vi "Data_raw-save.vi"(5 "timedelay":dbl[](array[numeric])=[0.0, 1.0, 2.0, 3.0, 4.0, 5.0, 6.0, 7.0, 8.0, 9.0], 6 "data value reference":refnum<data-value>, 7 "wavelength":dbl[](array[numeric])=[10.0, 20.0, 0.0, 0.0, 0.0, 0.0, 0.0, 0.0, 0.0, 0.0, 0.0, 0.0, 0.0, 0.0, 0.0, 0.0, 0.0, 0.0, 0.0, 0.0, 0.0, 0.0, 0.0, 0.0, 0.0, 0.0, 0.0, 0.0, 0.0, 0.0, 0.0, 0.0, 0.0, 0.0, 0.0, 0.0, 0.0, 0.0, 0.0, 0.0, 0.0, 0.0, 0.0, 0.0, 0.0, 0.0, 0.0, 0.0, 0.0, 0.0, 0.0, 0.0, 0.0, 0.0, 0.0, 0.0, 0.0, 0.0, 0.0, 0.0, 0.0, 0.0, 0.0, 0.0, 0.0, 0.0, 0.0, 0.0, 0.0, 0.0, 0.0, 0.0, 0.0, 0.0, 0.0, 0.0, 0.0, 0.0, 0.0, 0.0, 0.0, 0.0, 0.0, 0.0, 0.0, 0.0, 0.0, 0.0, 0.0, 0.0, 0.0, 0.0, 0.0, 0.0, 0.0, 0.0, 0.0, 0.0, 0.0, 100.0], 8 "error in":errorcluster, 9 "file (use dialog)":path=path "C:/Users/Sergey Denisov/Documents/REPS/TRANCON/test2.txt.txt", 10 "accuracy":string="%#g", 11 "Data raw":i32[][][][](array[numeric])) -> (0 "error out":errorcluster)   [LabVIEW 2015]
panel:
  out "Done":bool
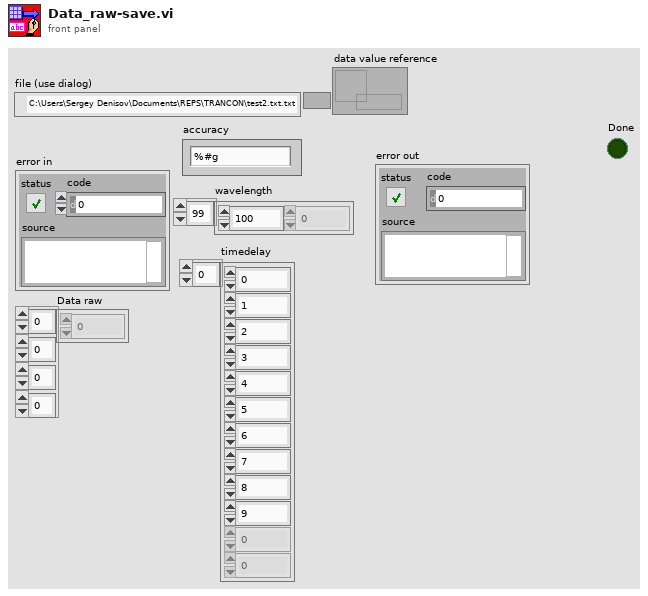
[diagram p1: front panel]
types:
  T1 = enum16{"open", "replace", "create", "open or create", "replace or create", "replace or create with confirmation"}
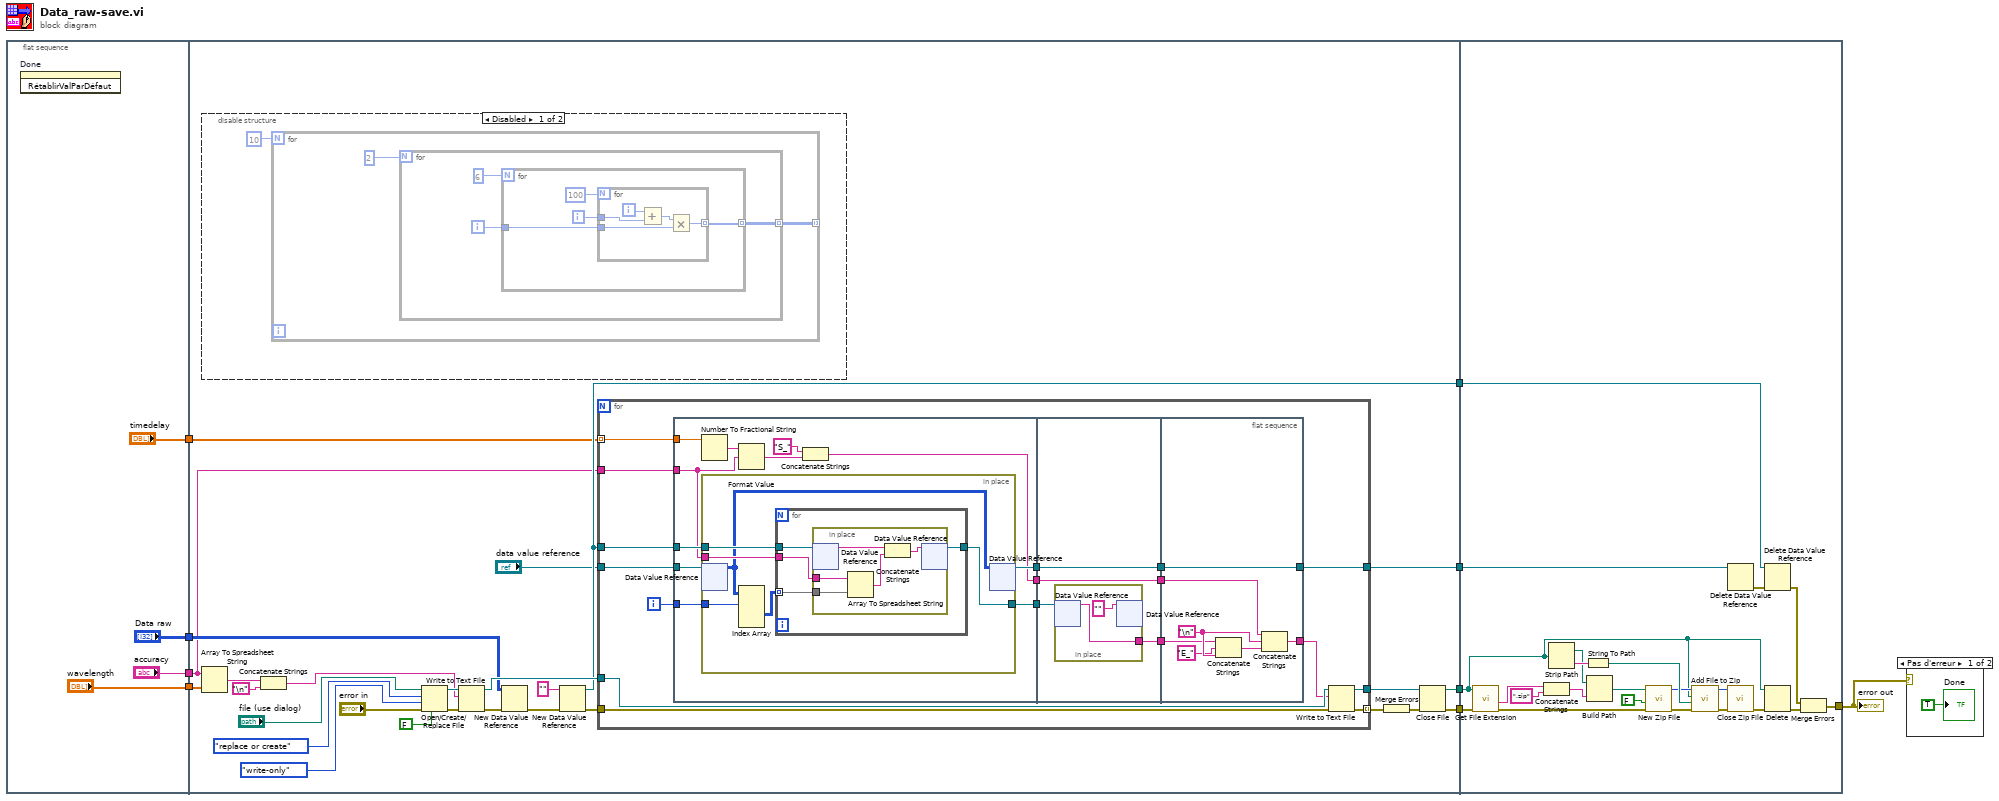
[diagram p0: block diagram]
diagram:
  n1 = flat-sequence {
    tunnel: ["Data raw"] -> w5
    tunnel: ["wavelength"] -> w4
    tunnel: ["timedelay"] -> w3
    tunnel: ["accuracy"] -> w2
    tunnel: [w24] -> w8
    tunnel: [w23] -> w7
    tunnel: [w22] -> w6
    tunnel: w5 -> [w21]
    tunnel: w4 -> [w18]
    tunnel: w3 -> [w17]
    tunnel: w2 -> [w16]
    tunnel: [w14] -> w1
    tunnel: w8 -> [w131]
    tunnel: w7 -> [w115]
    tunnel: w6 -> [w129]
    tunnel: [w133] -> w9
    tunnel: w1 -> [w113]
    frame #0 {
      n2 = invoke on="Done" class="Bool (strict)" method="RétablirValParDéfaut"() -> ()  [unwired: 3 in, 3 out]
    }
    frame #1 {
      n3 = disable-structure shown="Disabled" {
        frame Disabled {
          n4 = for {
            N: 10 -> [_]
            tunnel: [w43] -> _ mode=indexing
            n5 = for {
              N: 2 -> [_]
              tunnel: [w46] -> w43 mode=indexing
              i -> [w44]
              n6 = for {
                N: 6 -> [_]
                tunnel: [w50] -> w46 mode=indexing
                tunnel: w44 -> [w48]
                i -> [w47]
                n7 = for {
                  N: 100 -> [_]
                  tunnel: [w55] -> w50 mode=indexing
                  tunnel: w48 -> [w54]
                  tunnel: w47 -> [w51]
                  i -> [w53]
                  n8 = Add(x=w53, y=w51) -> (x+y=w52:i32)
                  n9 = Multiply(x=w52, y=w54) -> (x*y=w55:i32)
                }
              }
            }
          }
        }
        frame Enabled {
        }
      }
      n10 = Array To Spreadsheet String(array=w18, 3:w16) -> (spreadsheet string=w39:string)  [unwired: 1 in]
      n11 = Concatenate Strings(w39, "\n") -> (w29:string)
      n12 = Open/Create/Replace File(file path (use dialog)="file (use dialog)", error in="error in", operation (0:open)=T1."replace or create", access (0:read/write)=enum16{"read/write", "read-only", "write-only"}."write-only", disable buffering (F)=FALSE) -> (refnum out=w31:refnum<file>, error out=w28:errorcluster)  [unwired: 1 in, 1 out]
      n13 = Write to Text File(file (use dialog)=w31, text=w29, error in=w28) -> (refnum out=w30:refnum<file>, error out=w27:errorcluster)  [unwired: 1 in, 1 out]
      n14 = New Data Value Reference(data value=w21, error in=w27) -> (error out=w20:errorcluster)  [unwired: 1 out]
      n15 = New Data Value Reference(data value="" ("concatenated string"), error in=w20) -> (data value reference=w24:refnum<data-value>, error out=w19:errorcluster)
      n16 = for {
        tunnel: w17 -> [w59] mode=indexing
        tunnel: w16 -> [w72]
        tunnel: w30 -> [w68]
        tunnel: w19 -> [w63]
        tunnel: [w71] -> w26 mode=indexing
        tunnel: [w70] -> w36
        tunnel: w24 -> [w69]
        tunnel: "data value reference" -> [w67]
        tunnel: [w65] -> w22
        i -> [w56]
        n17 = flat-sequence {
          tunnel: w72 -> [w75]
          tunnel: w69 -> [w83]
          tunnel: w67 -> [w82]
          tunnel: [w81] -> w66
          tunnel: [w80] -> w64
          tunnel: w59 -> [w76]
          tunnel: [w74] -> w58
          tunnel: w56 -> [w73]
          tunnel: w66 -> [w102]
          tunnel: w64 -> [w100]
          tunnel: [w101] -> w62
          tunnel: [w100] -> w61
          tunnel: w58 -> [w99]
          tunnel: [w99] -> w57
          tunnel: [w111] -> w65
          tunnel: w62 -> [w105]
          tunnel: w61 -> [w111]
          tunnel: [w107] -> w60
          tunnel: w57 -> [w106]
          frame #0 {
            n18 = Number To Fractional String(number=w76) -> (F-format string=w77:string)  [unwired: 3 in]
            n19 = in-place {
              in-place-border: w75 -> [w89]
              in-place-border: w83 -> [w88]
              in-place-border: [w87] -> w81
              in-place-border: w73 -> [w86]
              n20 = in-place-dvr #1(w82) -> (w85:i32[][][][])  [unwired: 1 out]
              n21 = Index Array(array=w85, index (dim 0)=w86) -> (element=w84:i32[][][])  [unwired: 3 in]
              n22 = for {
                tunnel: w89 -> [w93]
                tunnel: w88 -> [w92]
                tunnel: w84 -> [w91] mode=indexing
                tunnel: [w90] -> w87
                n23 = in-place {
                  in-place-border: w93 -> [w98]
                  in-place-border: w91 -> [w94]
                  n24 = in-place-dvr #2(w92) -> (w96:string)  [unwired: 1 out]
                  n25 = Array To Spreadsheet String(array=w94, 3:w98) -> (spreadsheet string=w97:string)  [unwired: 1 in]
                  n26 = Concatenate Strings(w96, w97) -> (w95:string)
                  n27 = in-place-dvr #2(w95) -> (w90:refnum<data-value>)  [unwired: 1 out]
                }
              }
              n28 = in-place-dvr #1(w85) -> (w80:refnum<data-value>)  [unwired: 1 out]
            }
            n29 = Format Value(string ("")=w77, format string=w75) -> (output string=w79:string)  [unwired: 1 in]
            n30 = Concatenate Strings("S_", w79) -> (w74:string)
          }
          frame #1 {
            n31 = in-place {
              in-place-border: [w103] -> w101
              n32 = in-place-dvr #3(w102) -> (w103:string)  [unwired: 1 out]
              n33 = in-place-dvr #3("" ("data value")) -> ()  [unwired: 2 out]
            }
          }
          frame #2 {
            w110 = "\n"
            n34 = Concatenate Strings(w105, "E_" ("string"), w110) -> (w108:string)
            n35 = Concatenate Strings(w106, w110, w108) -> (w107:string)
          }
        }
        n36 = Write to Text File(file (use dialog)=w68, text=w60, error in=w63) -> (refnum out=w70:refnum<file>, error out=w71:errorcluster)  [unwired: 1 in, 1 out]
      }
      n37 = Merge Errors(w26) -> (w37:errorcluster)
      n38 = Close File(refnum=w36, error in=w37) -> (path=w14:path, error out=w23:errorcluster)
    }
    frame #2 {
      n39 = call <vilib>:"Get File Extension.vi"("error in (no error)"=w115, "file"=w113) -> ("error out"=w125:errorcluster, "filename without extension"=w126:string)  [unwired: 5 in, 3 out]
      n40 = Concatenate Strings(w126, ".zip" ("string")) -> (w124:string)
      n41 = Strip Path(path=w113) -> (stripped path=w116:path, name=w127:string)
      n42 = String To Path(string=w127) -> (path=w128:path)
      n43 = Build Path(base path=w116, name or relative path=w124) -> (appended path=w123:path)
      n44 = call <vilib>:"New Zip File.vi"("error in (no error)"=w125, "confirm overwrite? (F)"=FALSE, "target"=w123) -> ("error out"=w119:errorcluster, "zip file out"=w118:i64)  [unwired: 2 in, 1 out]
      n45 = call <vilib>:"Add File to Zip.vi"("error in (no error)"=w119, "destination path in zip"=w128, "source file path"=w113, "zip file in"=w118) -> ("error out"=w120:errorcluster, "zip file out"=w121:i64)  [unwired: 6 in]
      n46 = Delete Data Value Reference(data value reference=w129) -> (error out=w132:errorcluster)  [unwired: 1 in, 1 out]
      n47 = call <vilib>:"Close Zip File.vi"("error in (no error)"=w120, "zip file in"=w121) -> ("error out"=w114:errorcluster)  [unwired: 5 in]
      n48 = Delete Data Value Reference(data value reference=w131, error in=w132) -> (error out=w130:errorcluster)  [unwired: 1 out]
      n49 = Delete(path (use dialog)=w113, error in=w114) -> (error out=w112:errorcluster)  [unwired: 3 in, 2 out]
      n50 = Merge Errors(w130, w112) -> (w133:errorcluster)
    }
  }
  n51 = case shown="Pas d'erreur" w9 {
    frame No Error {
      "Done" <- TRUE ("Done")
    }
    frame Error {
    }
  }
  "error out" <- w9
